vi "Make_Tree_Item.vi"(8 "error in (no error)":errorcluster, 11 "IB_Source_Folder in":refnum<class "IB_Source_Folder.lvclass">) -> (0 "error out":errorcluster, 3 "TreeSrcItem":refnum<class "IB_Tree_Item_Source.lvclass">)   [LabVIEW 2020, in "IB_Source_Folder.lvclass"]
uses:
  <vilib>/AppBuilder/IB_Classes/Source/Container/Folder/IB_Source_Folder.lvclass
  <vilib>/AppBuilder/IB_Classes/Source/Container/Folder/IB_Source_Folder.lvclass/IB_Source_Folder.ctl
  <vilib>/AppBuilder/IB_Classes/Tree_Item_Source_Folder_Sync/IB_Tree_Item_Source_Folder_Sync.lvclass
  e:/builds/penguin/labview/branches/2020/dev/dist/vi.lib/AppBuilder/IB_Classes/Source/Container/IB_Source_Container.lvclass
  e:/builds/penguin/labview/branches/2020/dev/dist/vi.lib/AppBuilder/IB_Classes/Source/IB_Source.lvclass
  e:/builds/penguin/labview/branches/2020/dev/dist/vi.lib/AppBuilder/IB_Classes/Source/Container/Folder/IB_Source_Folder.lvclass
  e:/builds/penguin/labview/branches/2020/dev/dist/vi.lib/AppBuilder/IB_Classes/Tree_Item_Source_Folder/IB_Tree_Item_Source_Folder.lvclass
  e:/builds/penguin/labview/branches/2020/dev/dist/vi.lib/AppBuilder/IB_Classes/Tree_Item_Source_Container/IB_Tree_Item_Source_Container.lvclass
  e:/builds/penguin/labview/branches/2020/dev/dist/vi.lib/AppBuilder/IB_Classes/Tree_Item_Source/IB_Tree_Item_Source.lvclass
  e:/builds/penguin/labview/branches/2020/dev/dist/vi.lib/AppBuilder/IB_Classes/Tree_Item/IB_Tree_Item.lvclass
  e:/builds/penguin/labview/branches/2020/dev/dist/vi.lib/AppBuilder/IB_Classes/Tree_Item_Source_Folder_Sync/IB_Tree_Item_Source_Folder_Sync.lvclass
  <vilib>/AppBuilder/IB_Classes/Tree_Item_Source/IB_Tree_Item_Source.lvclass
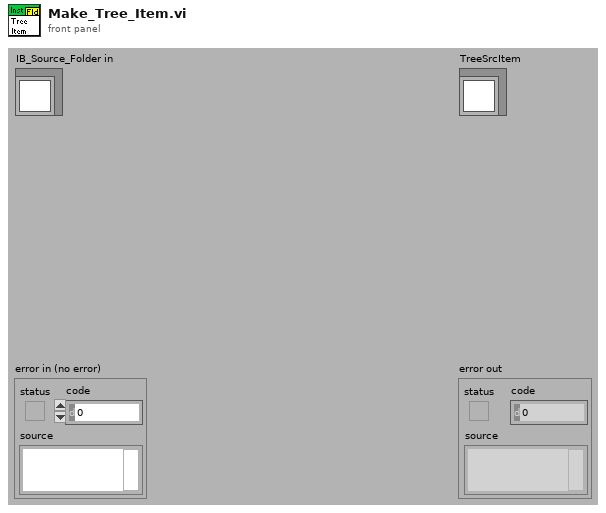
[diagram p1: front panel]
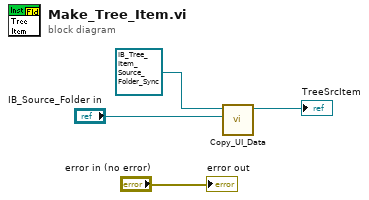
[diagram p0: block diagram]
diagram:
  n1 = call-dynamic "Copy_UI_Data.vi"("IB_Source in"="IB_Source_Folder in", "IB_TreeContainerItem.lvclass"=refnum<class "IB_Tree_Item_Source_Folder_Sync.lvclass"> refnum ("IB_TreeSyncFolderItem.lvclass")) -> ("IB_TreeContainerItem out"=→"TreeSrcItem":refnum<class "IB_Tree_Item_Source_Folder_Sync.lvclass">)  [unwired: 8 in, 1 out]
  "error out" <- "error in (no error)"
